vi "Report_Preview_Error.vi"(8 "error in (no error)":errorcluster, 11 "IB_Source_Container in":refnum<class "IB_Source_Container.lvclass">) -> (0 "error out":errorcluster, 3 "IB_Source_Container out":refnum<class "IB_Source_Container.lvclass">)   [LabVIEW 2020, in "IB_Source_Container.lvclass"]
uses:
  <vilib>/AppBuilder/IB_Classes/Source/Container/IB_Source_Container.lvclass
  <vilib>/AppBuilder/IB_Classes/Source/Container/IB_Source_Container.lvclass/IB_Source_Container.ctl
  <resource>/Framework/Providers/Builds/Installer/CDK_GLOBAL_STRINGS.vi
  <vilib>/AppBuilder/IB_Classes/Source/IB_Source.lvclass
  e:/builds/penguin/labview/branches/2020/dev/dist/vi.lib/AppBuilder/IB_Classes/Source/IB_Source.lvclass
  e:/builds/penguin/labview/branches/2020/dev/dist/vi.lib/AppBuilder/IB_Classes/Source/Container/IB_Source_Container.lvclass
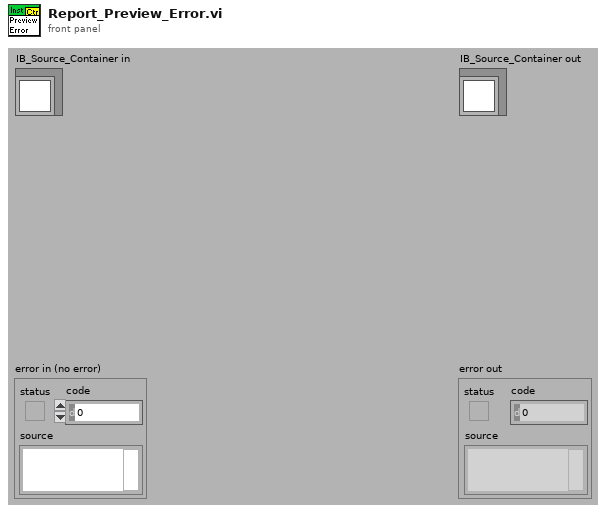
[diagram p1: front panel]
types:
  T1 = typedef "IB_Source.ctl" = cluster{"name":string, "sourceTag":string, "destTag":string, "path":path, "eng_installPath":string, "UI_inBuild?":bool, "str ref?":bool}
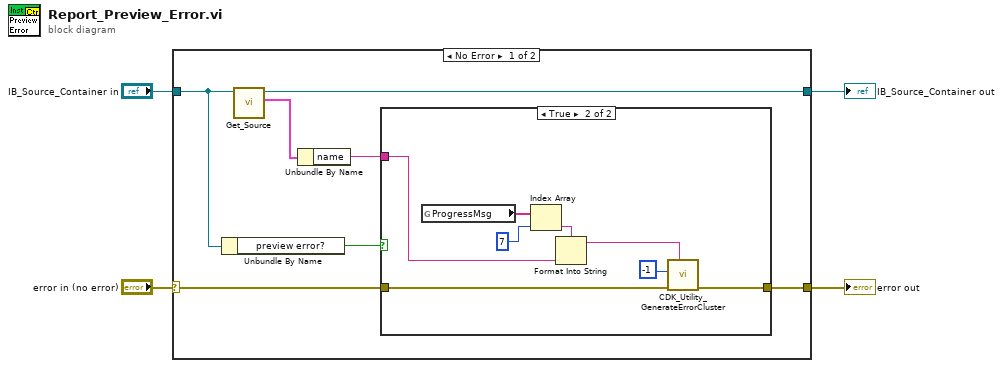
[diagram p0: block diagram]
diagram:
  n1 = case shown="No Error" "error in (no error)" {
    selector: "error in (no error)" -> [w10 w22]
    tunnel: [w9 w22] -> w3
    tunnel: "IB_Source_Container in" -> [w8 w21]
    tunnel: [w7 w21] -> w1
    frame No Error {
      n2 = Unbundle By Name(w8) -> ("preview error?"=w11:bool)
      n3 = call <vilib>:"Get_Source.vi"("IB_Source in"=w8) -> ("data"=w6:T1, "IB_Source out"=w7:refnum<class "IB_Source_Container.lvclass">)  [unwired: 1 in, 8 out]
      n4 = Unbundle By Name(w6) -> ("name"=w5:string)
      n5 = case shown="True" w11 {
        tunnel: w10 -> [w12 w17]
        tunnel: [w12 w16] -> w9
        tunnel: w5 -> [_ w13]
        frame False {
        }
        frame True {
          n6 = global read "CDK_GLOBAL_STRINGS.vi" "ProgressMsg"() -> (w20:string[])
          n7 = Index Array(array=w20, index=7) -> (element=w15:string)
          n8 = Format Into String(format string=w15, w13) -> (resulting string=w14:string)  [unwired: 2 in, 1 out]
          n9 = call <resource>:"CDK_Utility_GenerateErrorCluster.vi"("Additional Info"=w14, "ErrIn"=w17, "code"=-1) -> ("ErrOut"=w16:errorcluster)  [unwired: 1 in, 7 out]
        }
      }
    }
    frame Error {
    }
  }
  "error out" <- w3
  "IB_Source_Container out" <- w1
